vi "Powerstage_Digital_in_v1.vi"() -> ()   [LabVIEW 2022 SP3]
uses:
  <vilib>/Instr/_visa.llb/VISA Flush IO Buffer Mask.ctl
  <vilib>/DAQmx/write.llb/DAQmx Write (Digital 1D Bool NChan 1Samp 1Line).vi
  <vilib>/DAQmx/miscellaneous.llb/DAQmx Fill In Error Info.vi
panel:
  out "Array":string[](array[string])
  out "error out":errorcluster
  in  "error in (no error)":errorcluster
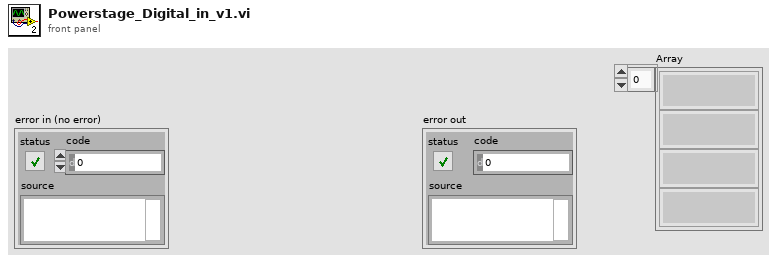
[diagram p1: front panel]
types:
  T1 = cluster{"State":string, "State off":string, "Vout":bool[], "Voff":bool[]}[]
  T2 = typedef "VISA Flush IO Buffer Mask.ctl" = u16
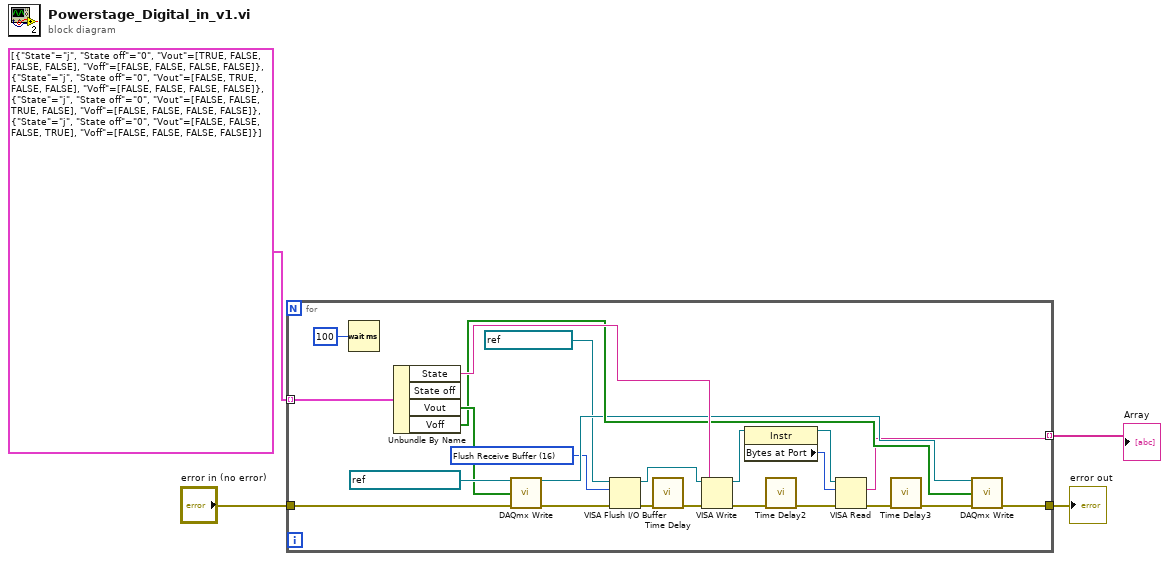
[diagram p0: block diagram]
diagram:
  n1 = for {
    tunnel: T1 [{"State"="j", "State off"="0", "Vout"=[TRUE, FALSE, FALSE, FALSE], "Voff"=[FALSE, FALSE, FALSE, FALSE]}, {"State"="j", "State off"="0", "Vout"=[FALSE, TRUE, FALSE, FALSE], "Voff"=[FALSE, FALSE, FALSE, FALSE]}, {"State"="j", "State off"="0", "Vout"=[FALSE, FALSE, TRUE, FALSE], "Voff"=[FALSE, FALSE, FALSE, FALSE]}, {"State"="j", "State off"="0", "Vout"=[FALSE, FALSE, FALSE, TRUE], "Voff"=[FALSE, FALSE, FALSE, FALSE]}] -> [w27] mode=indexing
    tunnel: "error in (no error)" -> [w22]
    tunnel: [w16] -> w2
    tunnel: [w5] -> w1 mode=indexing
    w8 = T2 16 items=["Flush Receive Buffer"=16, "Write Transmit Buffer to Device"=32, "Flush Receive Buffer (No I/O)"=64, "Flush Transmit Buffer"=128] ("Mask")
    n2 = Wait (ms)(milliseconds to wait=u32 100) -> ()  [unwired: 1 out]
    n3 = Unbundle By Name(w27) -> ("State"=w25:string, "Vout"=w20:bool[], "Voff"=w15:bool[])  [unwired: 1 out]
    n4 = call-poly <vilib>:"DAQmx Write.vi"("task/channels in"=refnum<k21> "FTS2_DigitalOut", "data"=w20, "error in"=w22) -> ("task out"=w14:refnum<k21>, "error out"=w6:errorcluster)  [unwired: 10 in, 1 out]
    n5 = VISA Flush I/O Buffer(VISA resource name=refnum<visa-resource-name> "ControlBoard", mask (16)=w8, error in (no error)=w6) -> (VISA resource name out=w10:refnum<visa-resource-name>, error out=w7:errorcluster)
    n6 = call "Time Delay"("error in (no error)"=w7) -> ("error out"=w24:errorcluster)  [unwired: 10 in]
    n7 = VISA Write(VISA resource name=w10, write buffer=w25, error in (no error)=w24) -> (VISA resource name out=w13:refnum<visa-resource-name>, error out=w23:errorcluster)  [unwired: 1 out]
    n8 = property class="Instr"(reference=w13) -> (reference out=w12:refnum<visa-resource-name>, "Bytes at Port"=w11:u32)  [unwired: 1 in, 1 out]
    n9 = call "Time Delay2"("error in (no error)"=w23) -> ("error out"=w19:errorcluster)  [unwired: 10 in]
    n10 = VISA Read(VISA resource name=w12, byte count=w11, error in (no error)=w19) -> (read buffer=w5:string, error out=w18:errorcluster)  [unwired: 2 out]
    n11 = call "Time Delay3"("error in (no error)"=w18) -> ("error out"=w17:errorcluster)  [unwired: 10 in]
    n12 = call-poly <vilib>:"DAQmx Write.vi"("task/channels in"=w14, "data"=w15, "error in"=w17) -> ("error out"=w16:errorcluster)  [unwired: 10 in, 2 out]
  }
  "error out" <- w2
  "Array" <- w1
